vi "Example4- Times.vi"() -> ()   [LabVIEW 2020]
doc: "Shows time diference between passing data with four method: by wire, local variable, direct property node and property node by refefernce."
panel:
  out "Time 4":dbl format="%.6f"
  out "Time 3":dbl format="%.6f"
  out "Time 2":dbl format="%.6f"
  out "Time1":dbl format="%.6f"
  in  "Numeric 3":i64
  out "Numeric 1 Out":i64
  in  "Numeric 2":i64
  in  "Numeric 4":i64
  in  "Numeric 1":i64
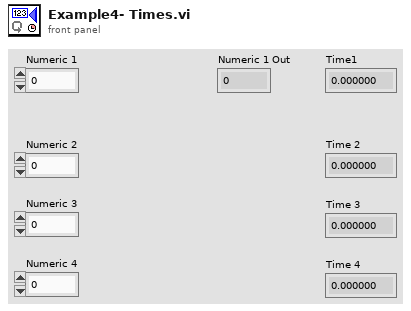
[diagram p1: front panel]
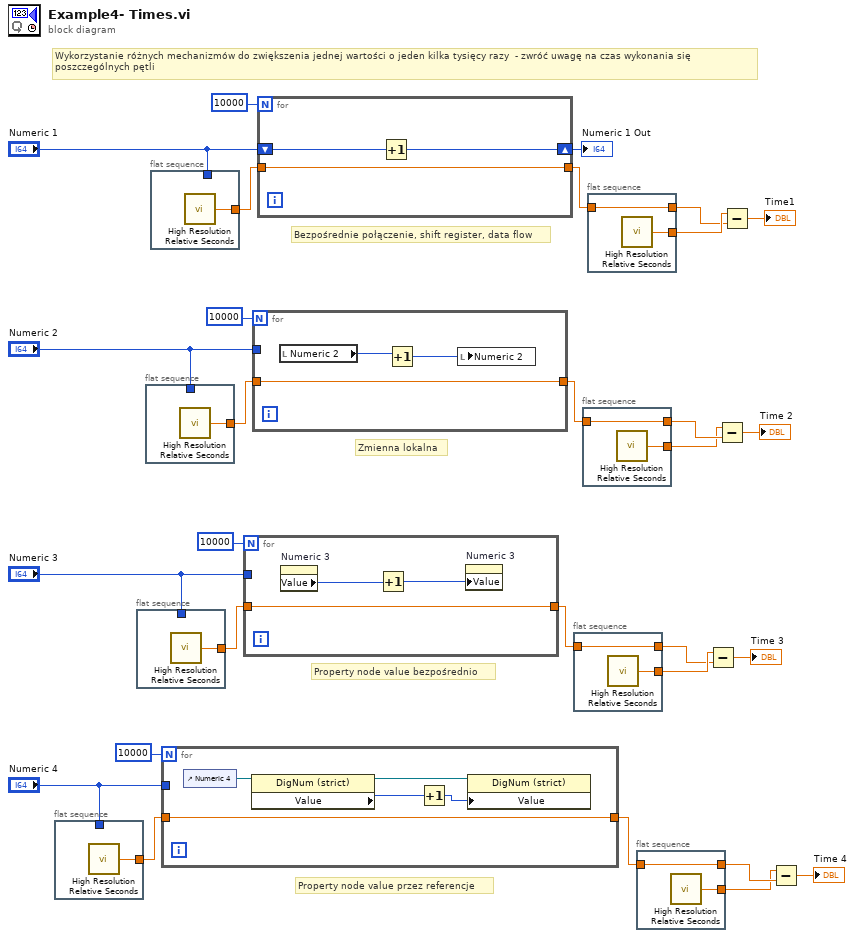
[diagram p0: block diagram]
diagram:
  # "Property node value przez referencje"
  # "Property node value bezpośrednio"
  # "Zmienna lokalna"
  # "Bezpośrednie połączenie, shift register, data flow"
  # "Wykorzystanie różnych mechanizmów do zwiększenia jednej wartości o jeden kilka tysięcy razy  - zwróć uwagę na czas wykonania się \nposzczególnych pętli"
  n1 = flat-sequence {
    tunnel: [w30] -> w3
    tunnel: "Numeric 4" -> [_]
    frame #0 {
      n2 = call <vilib>:"High Resolution Relative Seconds.vi"() -> ("relative seconds"=w30:dbl)
    }
  }
  n3 = flat-sequence {
    tunnel: [w31] -> w13
    tunnel: "Numeric 3" -> [_]
    frame #0 {
      n4 = call <vilib>:"High Resolution Relative Seconds.vi"() -> ("relative seconds"=w31:dbl)
    }
  }
  n5 = flat-sequence {
    tunnel: [w32] -> w17
    tunnel: "Numeric 2" -> [_]
    frame #0 {
      n6 = call <vilib>:"High Resolution Relative Seconds.vi"() -> ("relative seconds"=w32:dbl)
    }
  }
  n7 = flat-sequence {
    tunnel: "Numeric 1" -> [_]
    tunnel: [w33] -> w26
    frame #0 {
      n8 = call <vilib>:"High Resolution Relative Seconds.vi"() -> ("relative seconds"=w33:dbl)
    }
  }
  n9 = for {
    N: 10000 -> [_]
    tunnel: w3 -> [w38]
    tunnel: [w38] -> w4
    tunnel: "Numeric 4" -> [_]
    n10 = control-ref of="Numeric 4"() -> (w37:refnum<vi>)
    n11 = property class="DigNum (strict)"(reference=w37) -> (reference out=w35:refnum<vi>, "Value"=w36:i64)  [unwired: 1 in, 1 out]
    n12 = Increment(x=w36) -> (x+1=w34:i64)
    n13 = property class="DigNum (strict)"(reference=w35, "Value"=w34) -> ()  [unwired: 1 in, 2 out]
  }
  n14 = for {
    N: 10000 -> [_]
    tunnel: w13 -> [w41]
    tunnel: [w41] -> w12
    tunnel: "Numeric 3" -> [_]
    n15 = property on="Numeric 3" class="DigNum (strict)"() -> ("Value"=w40:i64)  [unwired: 2 in, 2 out]
    n16 = Increment(x=w40) -> (x+1=w39:i64)
    n17 = property on="Numeric 3" class="DigNum (strict)"("Value"=w39) -> ()  [unwired: 2 in, 2 out]
  }
  n18 = for {
    N: 10000 -> [_]
    tunnel: w17 -> [w44]
    tunnel: [w44] -> w18
    tunnel: "Numeric 2" -> [_]
    n19 = local read "Numeric 2"() -> (w43:i64)
    n20 = Increment(x=w43) -> (x+1=w42:i64)
    n21 = local write "Numeric 2"(w42) -> ()
  }
  n22 = for {
    N: 10000 -> [_]
    shift-right: [w46] -> w28
    shift-left: "Numeric 1" -> [w47]
    tunnel: w26 -> [w45]
    tunnel: [w45] -> w25
    n23 = Increment(x=w47) -> (x+1=w46:i64)
  }
  "Numeric 1 Out" <- w28
  n24 = flat-sequence {
    tunnel: [w49] -> w11
    tunnel: w12 -> [w48]
    tunnel: [w48] -> w10
    frame #0 {
      n25 = call <vilib>:"High Resolution Relative Seconds.vi"() -> ("relative seconds"=w49:dbl)
    }
  }
  n26 = flat-sequence {
    tunnel: [w51] -> w19
    tunnel: w18 -> [w50]
    tunnel: [w50] -> w20
    frame #0 {
      n27 = call <vilib>:"High Resolution Relative Seconds.vi"() -> ("relative seconds"=w51:dbl)
    }
  }
  n28 = flat-sequence {
    tunnel: [w53] -> w24
    tunnel: w25 -> [w52]
    tunnel: [w52] -> w23
    frame #0 {
      n29 = call <vilib>:"High Resolution Relative Seconds.vi"() -> ("relative seconds"=w53:dbl)
    }
  }
  n30 = flat-sequence {
    tunnel: [w55] -> w5
    tunnel: w4 -> [w54]
    tunnel: [w54] -> w6
    frame #0 {
      n31 = call <vilib>:"High Resolution Relative Seconds.vi"() -> ("relative seconds"=w55:dbl)
    }
  }
  n32 = Subtract(x=w11, y=w10) -> (x-y=→"Time 3":dbl)
  n33 = Subtract(x=w19, y=w20) -> (x-y=→"Time 2":dbl)
  n34 = Subtract(x=w24, y=w23) -> (x-y=→"Time1":dbl)
  n35 = Subtract(x=w5, y=w6) -> (x-y=→"Time 4":dbl)
